vi "Read New FIFO Publisher.vi"(8 "error in":errorcluster, 11 "ChanMngOOB_Tx in":refnum<class "ChnMngOOB_Tx.lvclass">) -> (0 "error out":errorcluster, 2 "FIFO Publisher":T1, 3 "ChanMngOOB_Tx out":refnum<class "ChnMngOOB_Tx.lvclass">)   [LabVIEW 2021, in "ChnMngOOB_Tx.lvclass"]
uses:
  ChnMngOOB_Tx.lvclass
  C:/Program Files/National Instruments/LabVIEW 2021/vi.lib/CIF Foundation/CIF Out of Band Commands/CIFOutOfBand.lvclass
  Typedef/FIFO Publisher Return.ctl
  <vilib>/CIF Foundation/CIF Out of Band Commands/CIFOutOfBand.lvclass/CIFOutOfBand.ctl
  <vilib>/CIF Foundation/CIF Out of Band Commands/Accessors/Read Local OOB Data.vi
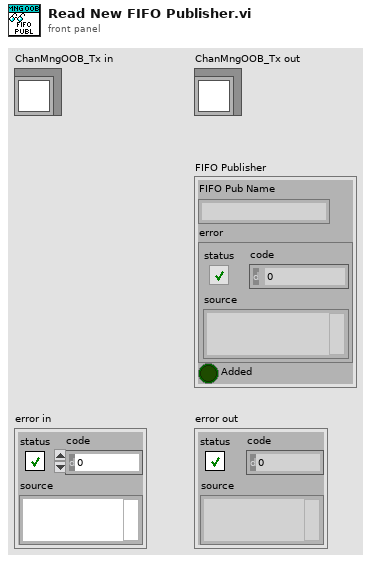
[diagram p1: front panel]
types:
  T1 = typedef "ChnMngOOB_Tx.lvclass/FIFO Publisher Return.ctl" = cluster{"FIFO Pub Name":string, "error":errorcluster, "Added":bool}
  T2 = typedef "ChnMngOOB_Tx.lvclass/Template Payload.ctl" = cluster{"Channel List":T3[], "New FIFO Publisher":T1}
  T3 = typedef "CIFChannelMng.lvclass/Channel List for OOB.ctl" = cluster{"Name":string, "Direction":T4, "Type":string, "Connected?":bool, "Connected Name":string, "Custom Config Data":u8[], "Forced?":bool}
  T4 = typedef "CIFChannels.lvclass/Direction.ctl" = enum16{"Publisher", "Subscriber"}
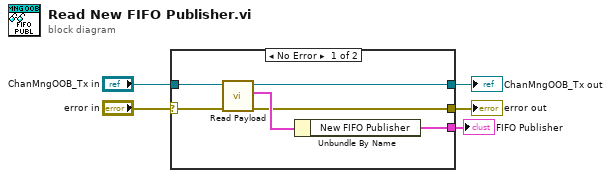
[diagram p0: block diagram]
diagram:
  n1 = case shown="No Error" "error in" {
    selector: "error in" -> [w7 w12]
    tunnel: [w6 w12] -> w4
    tunnel: [w10 w13] -> w2
    tunnel: "ChanMngOOB_Tx in" -> [w11 w13]
    tunnel: [w8 _] -> w1
    frame No Error {
      n2 = call "Read Payload.vi"("error in"=w7, "ChanMngOOB_Tx in"=w11) -> ("error out"=w6:errorcluster, "data"=w9:T2, "ChanMngOOB_Tx out"=w10:refnum<class "ChnMngOOB_Tx.lvclass">)  [unwired: 7 in]
      n3 = Unbundle By Name(w9) -> ("New FIFO Publisher"=w8:T1)
    }
    frame Error {
    }
  }
  "error out" <- w4
  "ChanMngOOB_Tx out" <- w2
  "FIFO Publisher" <- w1
